vi "get output data from library.vi"(8 "error in":errorcluster, 11 "lvsocket":u64) -> (0 "error out":errorcluster, 2 "data":string, 3 "err":i32)   [LabVIEW 2016, in "lv tls dll.lvlib"]
uses:
  lv tls dll.lvlib
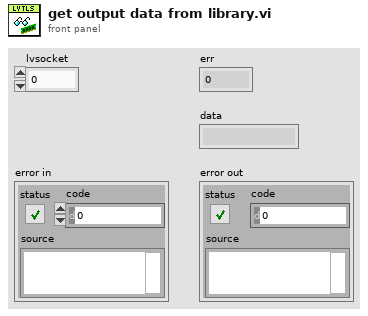
[diagram p1: front panel]
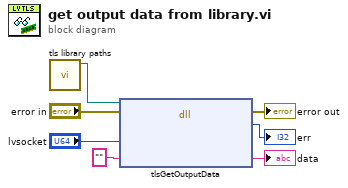
[diagram p0: block diagram]
diagram:
  n1 = call "tls library paths.vi"() -> ("lvtls"=w7:path)  [unwired: 8 in, 3 out]
  n2 = dll-call lib="C:/Users/IEUser/Desktop/tlssimple/lvlibtls.dll" fn="tlsGetOutputData"(path in=w7, error in="error in", "lvsocket"="lvsocket", "data"="") -> (error out=→"error out":errorcluster, "err"=→"err":i32, "data"=→"data":string)  [unwired: 2 in, 1 out]
